vi "LUTMode.vi"(6 "SetpParams":T1, 7 "Mode":u16(ring) items=["Get&Set", "Get", "Set"], 8 "Error_In":T2, 9 "NewLUTMode":u32, 10 "ChildNo":u32, 11 "DeviceNo":u32) -> (0 "Error_Out":T2, 2 "LUTMode":u32, 3 "Error?":bool, 4 "GetpParams":T1, 5 "LUTModeList":cluster{string, i32}[](array[cluster]))   [LabVIEW 2015]
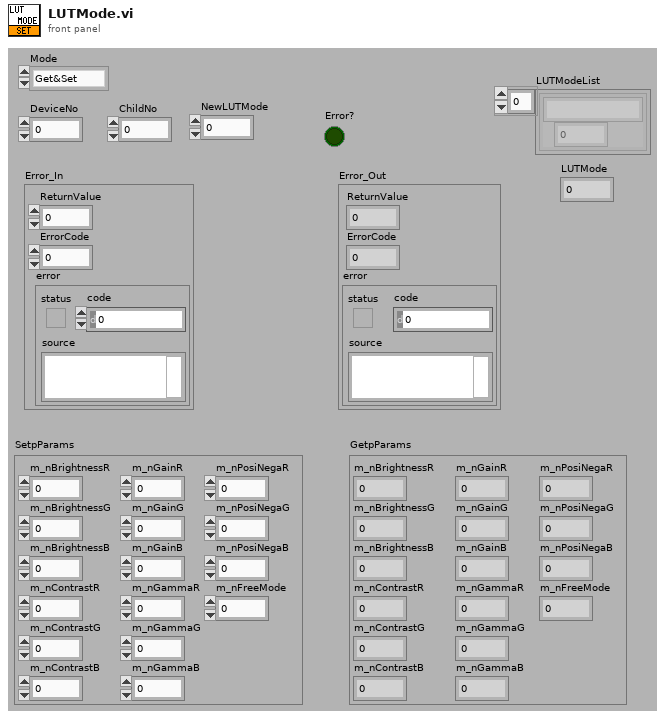
[diagram p1: front panel]
types:
  T1 = cluster{"m_nBrightnessR":i32, "m_nBrightnessG":i32, "m_nBrightnessB":i32, "m_nContrastR":i32, "m_nContrastG":i32, "m_nContrastB":i32, "m_nGainR":dbl, "m_nGainG":dbl, "m_nGainB":dbl, "m_nGammaR":dbl, "m_nGammaG":dbl, "m_nGammaB":dbl, "m_nPosiNegaR":u8, "m_nPosiNegaG":u8, "m_nPosiNegaB":u8, "m_nFreeMode":u8}
  T2 = cluster{"ReturnValue":u32, "ErrorCode":u32, "error ":errorcluster}
  T3 = cluster{"BrightnessR":i32, "BrightnessG":i32, "BrightnessB":i32, "ContrastR":i32, "ContrastG":i32, "ContrastB":i32, "GainR":dbl, "GainG":dbl, "GainB":dbl, "GammaR":dbl, "GammaG":dbl, "GammaB":dbl, "PosiNegaR":u8, "PosiNegaG":u8, "PosiNegaB":u8, "FreeMode":u8}
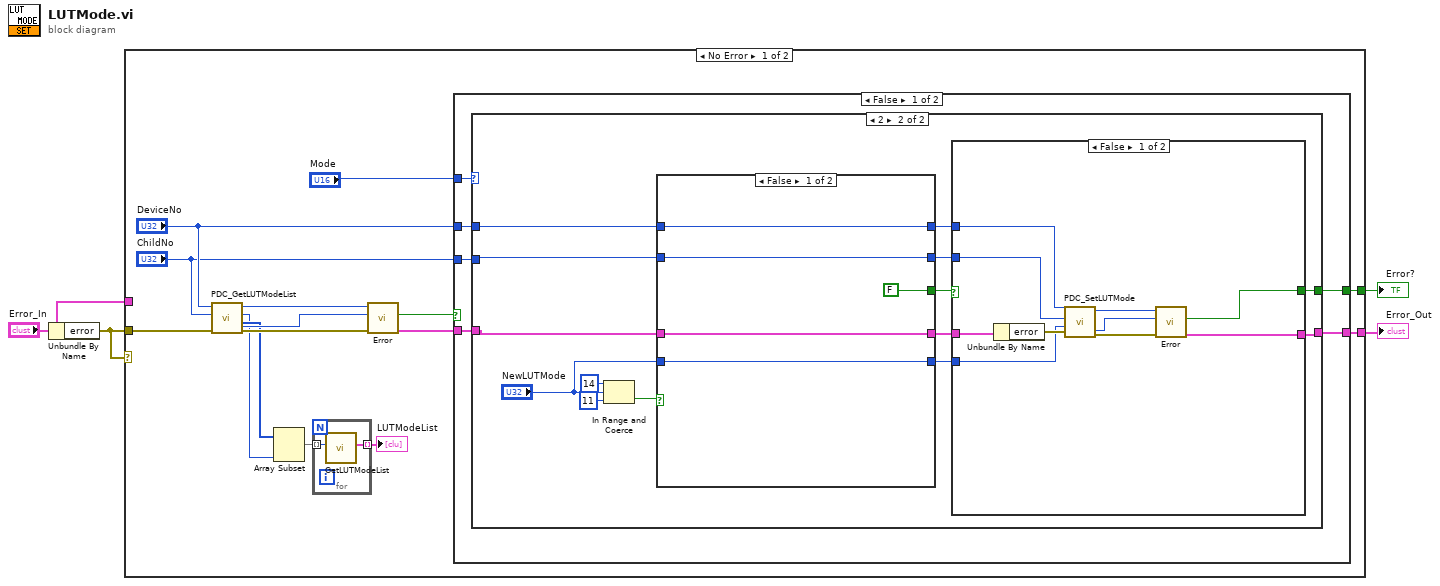
[diagram p0: block diagram]
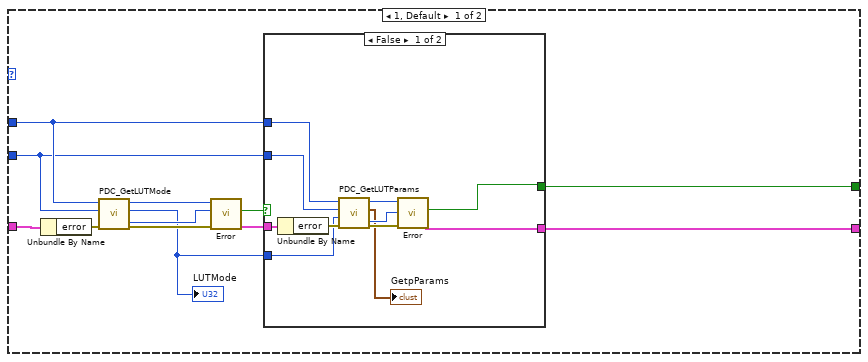
[diagram p2: hidden frame]
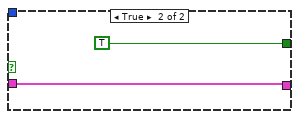
[diagram p3: hidden frame]
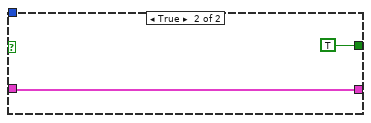
[diagram p4: hidden frame]
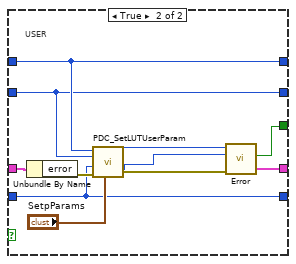
[diagram p5: hidden frame]
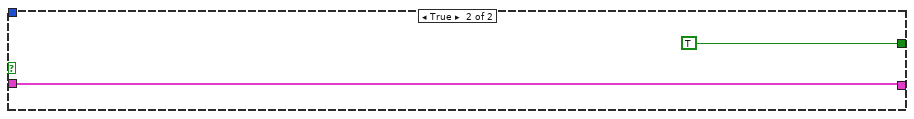
[diagram p6: hidden frame]
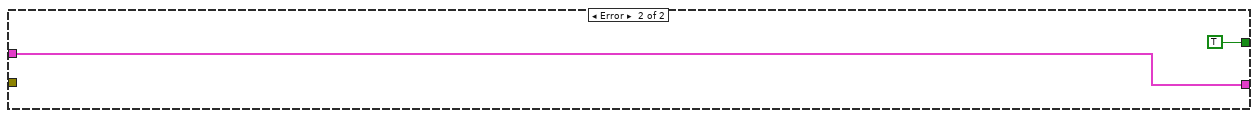
[diagram p7: hidden frame]
diagram:
  n1 = Unbundle By Name("Error_In") -> ("error"=w2:errorcluster)
  n2 = case shown="No Error" w2 {
    tunnel: [w19 w98] -> w4
    tunnel: [w18 TRUE ("Error?")] -> w3
    tunnel: w2 -> [w17 _]
    tunnel: "Error_In" -> [_ w98]
    frame No Error {
      n3 = call "PDC_GetLUTModeList.vi"("error in (no error)"=w17, "ChildNo"="ChildNo", "DeviceNo"="DeviceNo") -> ("error out"=w14:errorcluster, "List"=w8:u32[], "Size"=w7:u32, "ReturnValue"=w12:u32, "ErrorCode"=w11:u32)  [unwired: 4 out]
      n4 = Array Subset(array=w8, length=w7) -> (w9:u32[])  [unwired: 1 in]
      n5 = for {
        tunnel: w9 -> [w21] mode=indexing
        tunnel: [w20] -> w6 mode=indexing
        n6 = call "GetLUTModeList.vi"("List"=w21) -> ("GetLUTModeList"=w20:cluster{string, i32})  [unwired: 10 out]
      }
      "LUTModeList" <- w6
      n7 = call "Error.vi"("error in (no error)"=w14, "ErrorCode"=w11, "ReturnValue"=w12) -> ("Error_Out"=w13:T2, "Error?"=w10:bool)  [unwired: 7 out]
      n8 = case shown="False" w10 {
        tunnel: [w27 w96] -> w19
        tunnel: [w26 TRUE ("Error?")] -> w18
        tunnel: w13 -> [w25 w96]
        tunnel: "DeviceNo" -> [w24 _]
        tunnel: "ChildNo" -> [w23 _]
        tunnel: "Mode" -> [w22 _]
        frame False {
          n9 = case shown="2" w22 {
            tunnel: [w34 w57] -> w27
            tunnel: [w33 w53] -> w26
            tunnel: w25 -> [w30 w60]
            tunnel: w24 -> [w29 w65]
            tunnel: w23 -> [w28 w64]
            frame 1, Default {
              n10 = Unbundle By Name(w30) -> ("error"=w32:errorcluster)
              n11 = call "PDC_GetLUTMode.vi"("error in (no error)"=w32, "ChildNo"=w28, "DeviceNo"=w29) -> ("error out"=w37:errorcluster, "Mode"=w31:u32, "ReturnValue"=w38:u32, "ErrorCode"=w39:u32)  [unwired: 5 out]
              "LUTMode" <- w31
              n12 = call "Error.vi"("error in (no error)"=w37, "ErrorCode"=w39, "ReturnValue"=w38) -> ("Error_Out"=w35:T2, "Error?"=w36:bool)  [unwired: 7 out]
              n13 = case shown="False" w36 {
                tunnel: w35 -> [w50 w52]
                tunnel: [w41 w52] -> w34
                tunnel: w29 -> [w48 _]
                tunnel: w28 -> [w47 _]
                tunnel: [w40 TRUE ("Error?")] -> w33
                tunnel: w31 -> [w42 _]
                frame False {
                  n14 = Unbundle By Name(w50) -> ("error"=w49:errorcluster)
                  n15 = call "PDC_GetLUTParams.vi"("error in (no error)"=w49, "LUTMode"=w42, "ChildNo"=w47, "DeviceNo"=w48) -> ("error out"=w46:errorcluster, "Params"=→"GetpParams":T3, "ReturnValue"=w45:u32, "ErrorCode"=w44:u32)  [unwired: 4 out]
                  n16 = call "Error.vi"("error in (no error)"=w46, "ErrorCode"=w44, "ReturnValue"=w45) -> ("Error_Out"=w41:T2, "Error?"=w40:bool)  [unwired: 7 out]
                }
                frame True {
                }
              }
            }
            frame 2 {
              n17 = In Range and Coerce(upper limit=u32 14 ("上限"), x="NewLUTMode", lower limit=u32 11 ("下限")) -> (In Range?=w61:bool)  [unwired: 1 out]
              n18 = case shown="False" w61 {
                tunnel: [w82 w94] -> w58
                tunnel: [FALSE w91] -> w59
                tunnel: w65 -> [w81 w86]
                tunnel: w64 -> [w80 w85]
                tunnel: "NewLUTMode" -> [w79 w84]
                tunnel: w60 -> [w82 w87]
                tunnel: [w81 w86] -> w56
                tunnel: [w80 w85] -> w55
                tunnel: [w79 w84] -> w54
                frame False {
                }
                frame True {
                  # "USER"
                  n19 = Unbundle By Name(w87) -> ("error"=w92:errorcluster)
                  n20 = call "PDC_SetLUTUserParam.vi"("Params"="SetpParams", "error in (no error)"=w92, "LUTMode"=w84, "ChildNo"=w85, "DeviceNo"=w86) -> ("error out"=w93:errorcluster, "ReturnValue"=w90:u32, "ErrorCode"=w89:u32)  [unwired: 4 out]
                  n21 = call "Error.vi"("error in (no error)"=w93, "ErrorCode"=w89, "ReturnValue"=w90) -> ("Error_Out"=w94:T2, "Error?"=w91:bool)  [unwired: 7 out]
                }
              }
              n22 = case shown="False" w59 {
                tunnel: w58 -> [w72 w77]
                tunnel: [w71 w77] -> w57
                tunnel: w56 -> [w70 _]
                tunnel: w55 -> [w69 _]
                tunnel: w54 -> [w68 _]
                tunnel: [w67 TRUE ("Error?")] -> w53
                frame False {
                  n23 = Unbundle By Name(w72) -> ("error"=w76:errorcluster)
                  n24 = call "PDC_SetLUTMode.vi"("error in (no error)"=w76, "LUTMode"=w68, "ChildNo"=w69, "DeviceNo"=w70) -> ("error out"=w73:errorcluster, "ReturnValue"=w75:u32, "ErrorCode"=w74:u32)  [unwired: 5 out]
                  n25 = call "Error.vi"("error in (no error)"=w73, "ErrorCode"=w74, "ReturnValue"=w75) -> ("Error_Out"=w71:T2, "Error?"=w67:bool)  [unwired: 7 out]
                }
                frame True {
                }
              }
            }
          }
        }
        frame True {
        }
      }
    }
    frame Error {
    }
  }
  "Error_Out" <- w4
  "Error?" <- w3
